vi "midi-file_main.vi"() -> ()   [LabVIEW 2020]
uses:
  midi-file-event.midi/midi-file-event.midi.lvclass
  midi-file/MIDI Messages.ctl
  midi-file/Note Value.ctl
  midi-file-event.midi/midi-file-event.midi.lvclass/midi-file-event.midi.ctl
  midi-file-event.midi/Data1.get.vi
  midi-file-event.midi/MIDI_Messages.get.vi
  midi-file/midi-file.lvclass
  midi-file-events/midi-file-events.lvclass
panel:
  out "Array 2":T1[](array[typedef])
  out "Array 3":T2[](array[typedef])
  out "Array":dbl[](array[numeric])
  out "Track data by Track number":T3(c390)
  out "*(type *) &x 3":i16
  out "*(type *) &x 2":i32
  out "*(type *) &x":string
  out "subarray":u8[](array[numeric]) format="%.0x"
  in  "length":i32
  in  "index":i32
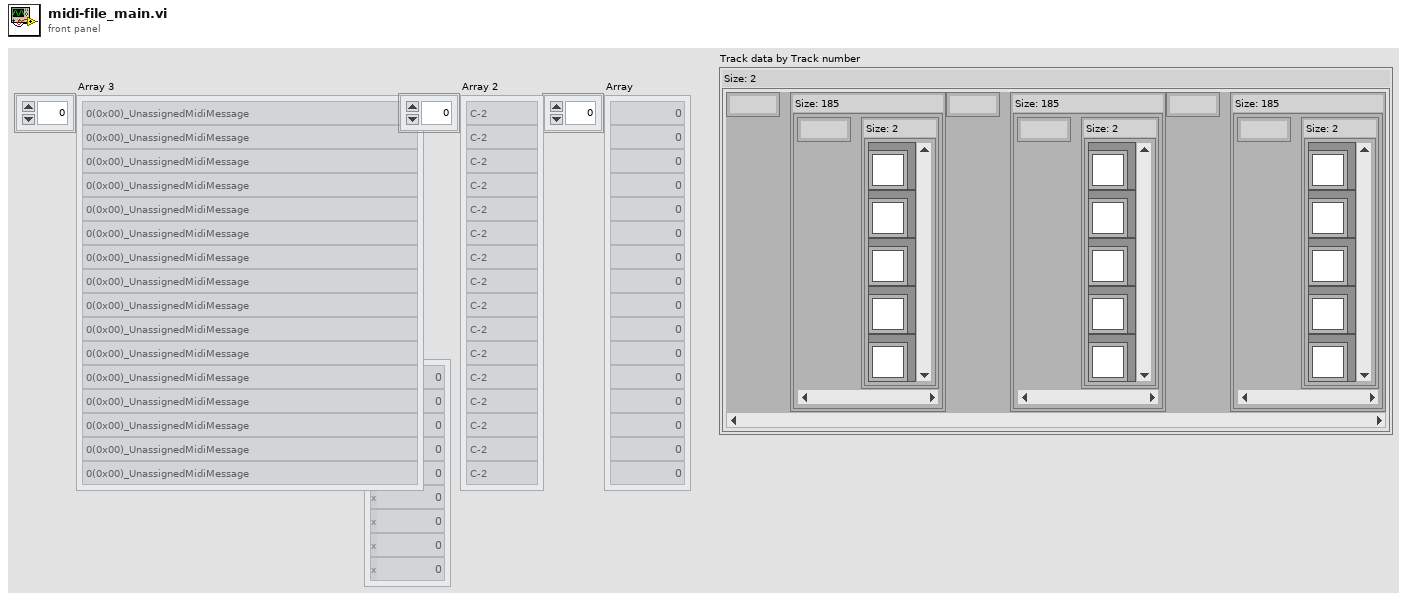
[diagram p1: front panel]
types:
  T1 = typedef "midi-file.lvclass/Note Value.ctl" = enum8{"C-2", "C#-2", "D-2", "D#-2", "E-2", "F-2", "F#-2", "G-2", "G#-2", "A-2", "A#-2", "B-2", "C-1", "C#-1", "D-1", "D#-1", "E-1", "F-1", "F#-1", "G-1", "G#-1", "A-1", "A#-1", "B-1", "C0", "C#0", "D0", "D#0", "E0", "F0", "F#0", "G0", "G#0", "A0", "A#0", "B0", "C1", "C#1", "D1", "D#1", "E1", "F1", "F#1", "G1", "G#1", "A1", "A#1", "B1", "C2", "C#2", "D2", "D#2", "E2", "F2", "F#2", "G2", "G#2", "A2", "A#2", "B2", "C3", "C#3", "D3", "D#3", "E3", "F3", "F#3", "G3", "G#3", "A3", "A#3", "B3", "C4", "C#4", "D4", "D#4", "E4", "F4", "F#4", "G4", "G#4", "A4", "A#4", "B4", "C5", "C#5", "D5", "D#5", "E5", "F5", "F#5", "G5", "G#5", "A5", "A#5", "B5", "C6", "C#6", "D6", "D#6", "E6", "F6", "F#6", "G6", "G#6", "A6", "A#6", "B6", "C7", "C#7", "D7", "D#7", "E7", "F7", "F#7", "G7", "G#7", "A7", "A#7", "B7", "C8", "C#8", "D8", "D#8", "E8", "F8", "F#8", "G"}
  T2 = typedef "midi-file.lvclass/MIDI Messages.ctl" = enum8{"0(0x00)_UnassignedMidiMessage", "1(0x01)_UnassignedMidiMessage", "2(0x02)_UnassignedMidiMessage", "3(0x03)_UnassignedMidiMessage", "4(0x04)_UnassignedMidiMessage", "5(0x05)_UnassignedMidiMessage", "6(0x06)_UnassignedMidiMessage", "7(0x07)_UnassignedMidiMessage", "8(0x08)_NoteOffEvent", "9(0x09)_NoteOnEvent", "10(0x0A)_PolyphonicKeyPressure", "11(0x0B)_ControlChange", "12(0x0C)_ProgramChange", "13(0x0D)_ChannelPressure", "14(0x0E)_PitchBendChange", "15(0x0F)_SystemExclusive(SysEx)", "16(0x10)_UnassignedMidiMessage", "17(0x11)_UnassignedMidiMessage", "18(0x12)_UnassignedMidiMessage", "19(0x13)_UnassignedMidiMessage", "20(0x14)_UnassignedMidiMessage", "21(0x15)_UnassignedMidiMessage", "22(0x16)_UnassignedMidiMessage", "23(0x17)_UnassignedMidiMessage", "24(0x18)_UnassignedMidiMessage", "25(0x19)_UnassignedMidiMessage", "26(0x1A)_UnassignedMidiMessage", "27(0x1B)_UnassignedMidiMessage", "28(0x1C)_UnassignedMidiMessage", "29(0x1D)_UnassignedMidiMessage", "30(0x1E)_UnassignedMidiMessage", "31(0x1F)_UnassignedMidiMessage", "32(0x20)_UnassignedMidiMessage", "33(0x21)_UnassignedMidiMessage", "34(0x22)_UnassignedMidiMessage", "35(0x23)_UnassignedMidiMessage", "36(0x24)_UnassignedMidiMessage", "37(0x25)_UnassignedMidiMessage", "38(0x26)_UnassignedMidiMessage", "39(0x27)_UnassignedMidiMessage", "40(0x28)_UnassignedMidiMessage", "41(0x29)_UnassignedMidiMessage", "42(0x2A)_UnassignedMidiMessage", "43(0x2B)_UnassignedMidiMessage", "44(0x2C)_UnassignedMidiMessage", "45(0x2D)_UnassignedMidiMessage", "46(0x2E)_UnassignedMidiMessage", "47(0x2F)_UnassignedMidiMessage", "48(0x30)_UnassignedMidiMessage", "49(0x31)_UnassignedMidiMessage", "50(0x32)_UnassignedMidiMessage", "51(0x33)_UnassignedMidiMessage", "52(0x34)_UnassignedMidiMessage", "53(0x35)_UnassignedMidiMessage", "54(0x36)_UnassignedMidiMessage", "55(0x37)_UnassignedMidiMessage", "56(0x38)_UnassignedMidiMessage", "57(0x39)_UnassignedMidiMessage", "58(0x3A)_UnassignedMidiMessage", "59(0x3B)_UnassignedMidiMessage", "60(0x3C)_UnassignedMidiMessage", "61(0x3D)_UnassignedMidiMessage", "62(0x3E)_UnassignedMidiMessage", "63(0x3F)_UnassignedMidiMessage", "64(0x40)_UnassignedMidiMessage", "65(0x41)_UnassignedMidiMessage", "66(0x42)_UnassignedMidiMessage", "67(0x43)_UnassignedMidiMessage", "68(0x44)_UnassignedMidiMessage", "69(0x45)_UnassignedMidiMessage", "70(0x46)_UnassignedMidiMessage", "71(0x47)_UnassignedMidiMessage", "72(0x48)_UnassignedMidiMessage", "73(0x49)_UnassignedMidiMessage", "74(0x4A)_UnassignedMidiMessage", "75(0x4B)_UnassignedMidiMessage", "76(0x4C)_UnassignedMidiMessage", "77(0x4D)_UnassignedMidiMessage", "78(0x4E)_UnassignedMidiMessage", "79(0x4F)_UnassignedMidiMessage", "80(0x50)_UnassignedMidiMessage", "81(0x51)_UnassignedMidiMessage", "82(0x52)_UnassignedMidiMessage", "83(0x53)_UnassignedMidiMessage", "84(0x54)_UnassignedMidiMessage", "85(0x55)_UnassignedMidiMessage", "86(0x56)_UnassignedMidiMessage", "87(0x57)_UnassignedMidiMessage", "88(0x58)_UnassignedMidiMessage", "89(0x59)_UnassignedMidiMessage", "90(0x5A)_UnassignedMidiMessage", "91(0x5B)_UnassignedMidiMessage", "92(0x5C)_UnassignedMidiMessage", "93(0x5D)_UnassignedMidiMessage", "94(0x5E)_UnassignedMidiMessage", "95(0x5F)_UnassignedMidiMessage", "96(0x60)_UnassignedMidiMessage", "97(0x61)_UnassignedMidiMessage", "98(0x62)_UnassignedMidiMessage", "99(0x63)_UnassignedMidiMessage", "100(0x64)_UnassignedMidiMessage", "101(0x65)_UnassignedMidiMessage", "102(0x66)_UnassignedMidiMessage", "103(0x67)_UnassignedMidiMessage", "104(0x68)_UnassignedMidiMessage", "105(0x69)_UnassignedMidiMessage", "106(0x6A)_UnassignedMidiMessage", "107(0x6B)_UnassignedMidiMessage", "108(0x6C)_UnassignedMidiMessage", "109(0x6D)_UnassignedMidiMessage", "110(0x6E)_UnassignedMidiMessage", "111(0x6F)_UnassignedMidiMessage", "112(0x70)_UnassignedMidiMessage", "113(0x71)_UnassignedMidiMessage", "114(0x72)_UnassignedMidiMessage", "115(0x73)_UnassignedMidiMessage", "116(0x74)_UnassignedMidiMessage", "117(0x75)_UnassignedMidiMessage", "118(0x76)_UnassignedMidiMessage", "119(0x77)_UnassignedMidiMessage", "120(0x78)_UnassignedMidiMessage", "121(0x79)_UnassignedMidiMessage", "122(0x7A)_UnassignedMidiMessage", "123(0x7B)_UnassignedMidiMessage", "124(0x7C)_UnassignedMidiMessage", "125(0x7D)_UnassignedMidiMessage", "126(0x7E)_UnassignedMidiMessage", "127(0x7F)_UnassignedMidiMessage"}
  T3 = map{i32, map{dbl, set{refnum<class "midi-file-event.midi.lvclass">}}}
  T4 = map{dbl, set{refnum<class "midi-file-event.midi.lvclass">}}
  T5 = set{refnum<class "midi-file-event.midi.lvclass">}
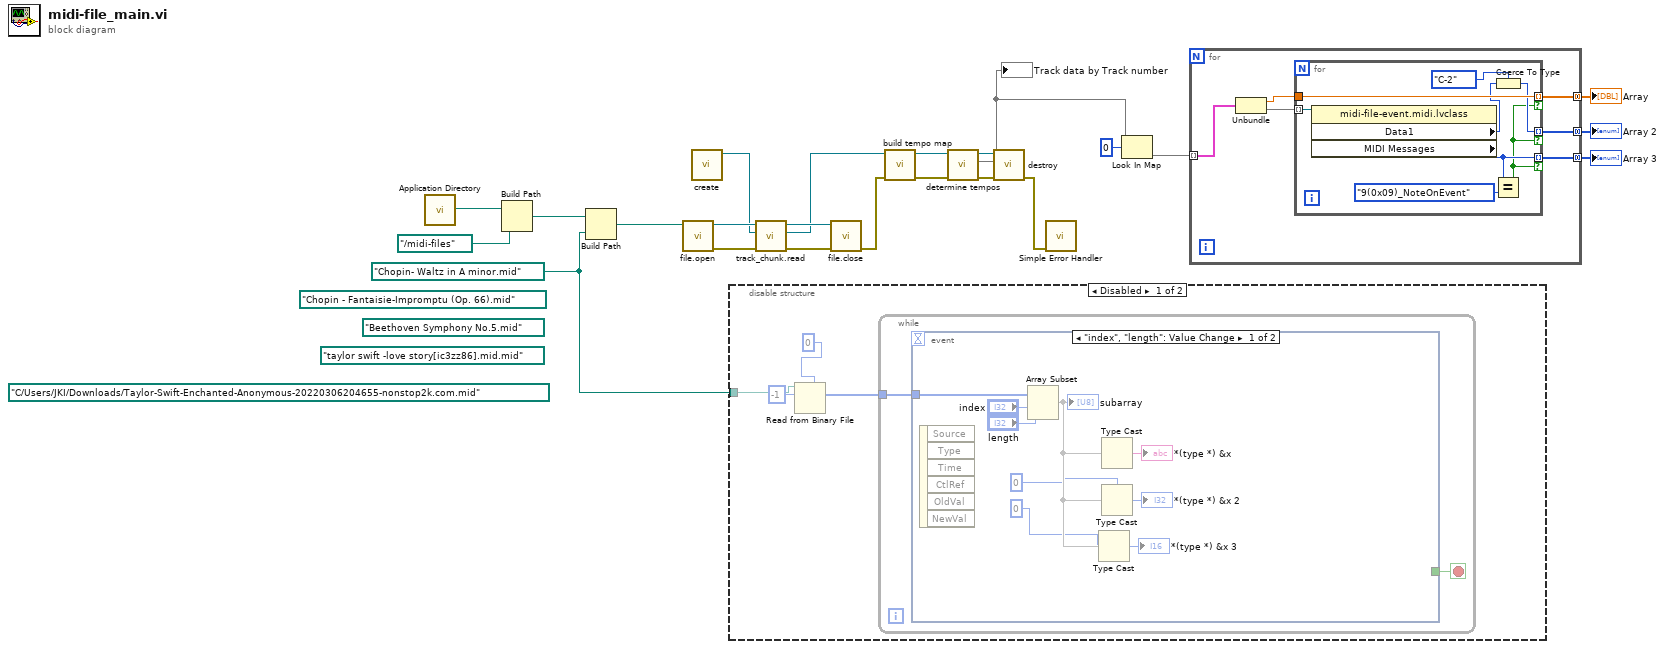
[diagram p0: block diagram]
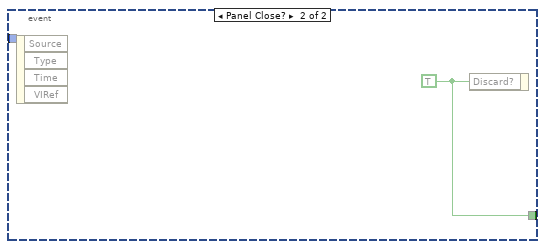
[diagram p2: hidden frame]
diagram:
  (unwired) path "C:/Users/JKI/Downloads/Taylor-Swift-Enchanted-Anonymous-20220306204655-nonstop2k.com.mid" ("Path to MIDI File (use dialog)")
  (unwired) path "taylor swift -love story[ic3zz86].mid.mid" ("Path to MIDI File (use dialog)")
  (unwired) path "Beethoven Symphony No.5.mid" ("Path to MIDI File (use dialog)")
  (unwired) path "Chopin - Fantaisie-Impromptu (Op. 66).mid" ("Path to MIDI File (use dialog)")
  w7 = path "Chopin- Waltz in A minor.mid" ("Path to MIDI File (use dialog)")
  n1 = call <vilib>:"Application Directory.vi"() -> ("Application Directory"=w23:path)
  n2 = Build Path(base path=w23, name or relative path=path "../midi-files") -> (appended path=w21:path)
  n3 = Build Path(base path=w21, name or relative path=w7) -> (appended path=w14:path)
  n4 = call "file.open.vi"("Path to MIDI File (use dialog)"=w14) -> ("error out"=w19:errorcluster, "midi-file out"=w20:refnum<class "midi-file.lvclass">)  [unwired: 9 in]
  n5 = call "create.vi"() -> ("midi-file-events"=w16:refnum<class "midi-file-events.lvclass">)  [unwired: 10 in, 1 out]
  n6 = disable-structure shown="Disabled" {
    disable-tunnel: w7 -> [w27 _]
    frame Disabled {
      n7 = Read from Binary File(5:u8 0, 10:-1 ("count (1)"), 11:w27) -> (2:w24:u8[])  [unwired: 3 in, 3 out]
      n8 = while {
        tunnel: w24 -> [w29]
        stop <- w28 stop-if-true
        n9 = event shown="[0] \"index\", \"length\": Value Change" {
          selector: _ -> [_ _]
          dyn-events: _ -> [_ _]
          timeout: _ -> [_ _]
          tunnel: w29 -> [w38 _]
          tunnel: [_ w39] -> w28
          event "index", "length": Value Change {
            n10 = event-data() -> ()  [unwired: 1 in, 6 out]
            n11 = Array Subset(array=w38, index="index", length="length") -> (w34:u8[])
            "subarray" <- w34
            n12 = Type Cast(type=i16 0, x=w34) -> (*(type *) &x=→"*(type *) &x 3":i16)
            n13 = Type Cast(x=w34) -> (*(type *) &x=→"*(type *) &x":string)  [unwired: 1 in]
            n14 = Type Cast(type=0, x=w34) -> (*(type *) &x=→"*(type *) &x 2":i32)
          }
          event Panel Close? {
            w39 = TRUE ("Discard?")
            n15 = event-data() -> ()  [unwired: 1 in, 4 out]
            n16 = event-data("Discard?"=w39) -> ()  [unwired: 1 in, 1 out]
          }
        }
      }
    }
    frame Enabled {
    }
  }
  n17 = call "track_chunk.read.vi"("error in"=w19, "midi-file-events in"=w16, "midi-file in"=w20) -> ("error out"=w18:errorcluster, "midi-file-events out"=w13:refnum<class "midi-file-events.lvclass">, "midi-file out"=w17:refnum<class "midi-file.lvclass">)  [unwired: 6 in]
  n18 = call "file.close.vi"("error in"=w18, "midi-file in"=w17) -> ("error out"=w15:errorcluster)  [unwired: 9 in]
  n19 = call "build tempo map.vi"("error in (no error)"=w15, "midi-file-events in"=w13) -> ("error out"=w10:errorcluster, "midi-file-events out"=w12:refnum<class "midi-file-events.lvclass">)  [unwired: 8 in]
  n20 = call "determine tempos.vi"("error in (no error)"=w10, "midi-file-events in"=w12) -> ("error out"=w9:errorcluster, "Track data by Track number"=w6:T3, "midi-file-events out"=w11:refnum<class "midi-file-events.lvclass">)  [unwired: 7 in]
  "Track data by Track number" <- w6
  n21 = call "destroy.vi"("error in (no error)"=w9, "midi-file-events"=w11) -> ("error out"=w8:errorcluster)  [unwired: 9 in]
  n22 = call <vilib>:"Simple Error Handler.vi"("error in (no error)"=w8) -> ()  [unwired: 4 in, 5 out]
  n23 = Look In Map(map=w6, key=0) -> (value=w4:T4)  [unwired: 1 in, 1 out]
  n24 = for {
    tunnel: w4 -> [w45] mode=indexing
    tunnel: [w43] -> w2 mode=concatenating
    tunnel: [w42] -> w1 mode=concatenating
    tunnel: [w40] -> w3 mode=concatenating
    n25 = Unbundle(w45) -> ("Timestamp"=w41:dbl, w44:T5)
    n26 = for {
      tunnel: w44 -> [w53] mode=indexing
      tunnel: [w48] -> w43 mode=indexing if=w46
      tunnel: [w50] -> w42 mode=indexing if=w46
      tunnel: [w52] -> w40 mode=indexing if=w46
      tunnel: w41 -> [w52]
      n27 = property class="midi-file-event.midi.lvclass"(reference=w53) -> ("Data1"=w51:u8, "MIDI Messages"=w48:T2)  [unwired: 1 in, 2 out]
      n28 = Coerce To Type(0:w51, 1:Note_Value."C-2" ("Note Value")) -> (2:w50:T1)
      n29 = Equal?(x=w48, y=MIDI_Messages."9(0x09)_NoteOnEvent") -> (x = y?=w46:bool)
    }
  }
  "Array" <- w3
  "Array 3" <- w2
  "Array 2" <- w1
